vi "Fluxo automatico.vi"() -> ()   [LabVIEW 2011]
uses:
  <vilib>/Utility/error.llb/DialogType.ctl
  <vilib>/Analysis/6fits.llb/Curve Fitting Criteria.ctl
  <vilib>/DAQmx/write.llb/DAQmx Write (Digital Bool 1Line 1Point).vi
  <vilib>/DAQmx/create/channels.llb/DAQmx Create Channel (DO-Digital Output).vi
  <vilib>/DAQmx/miscellaneous.llb/DAQmx Fill In Error Info.vi
  <vilib>/Analysis/NI_AALPro.lvlib
panel:
  out "P-manual":dynamicdata(graph)
  in  "stop":bool
  in  "path":path=path "C:/H2_Painel/painel_auto/cinetica.txt"
  out "Polynomial Coefficients":dbl[](array[numeric])
  in  "STOP carga":dbl=5.0
  out "error":i32
  out "intercept":dbl
  out "slope":dbl
  in  "Def P":dbl
  in  "SET number":i32
  out "Linear Model Graph":dbl[][](graph)
  in  "N fit":i32
  in  "precision (6)":i16=3
  out "T":bool
  out "ZPit":bool
  out "Pit":bool
  out "Pf2":bool
  out "ZPf2":bool
  out "String_cinetica":string
  in  "wait vacuo":u32=30000
  in  "ATM wait":u32
  out "Thermometer":dbl(slide) scale=0.0..30.0
  out "String":string
  out "Camara":dbl(slide) scale=0.0..20.0 scale format="%#_3g"
  out "Vácuo":bool
  out "Atm":bool
  out "Câmara":bool
  out "Vol Ref":dbl(slide) scale=0.0..10.0 scale format="%#_4f"
  out "Entrada gás":bool
  # "P vol ref"
  # "P Câmara"
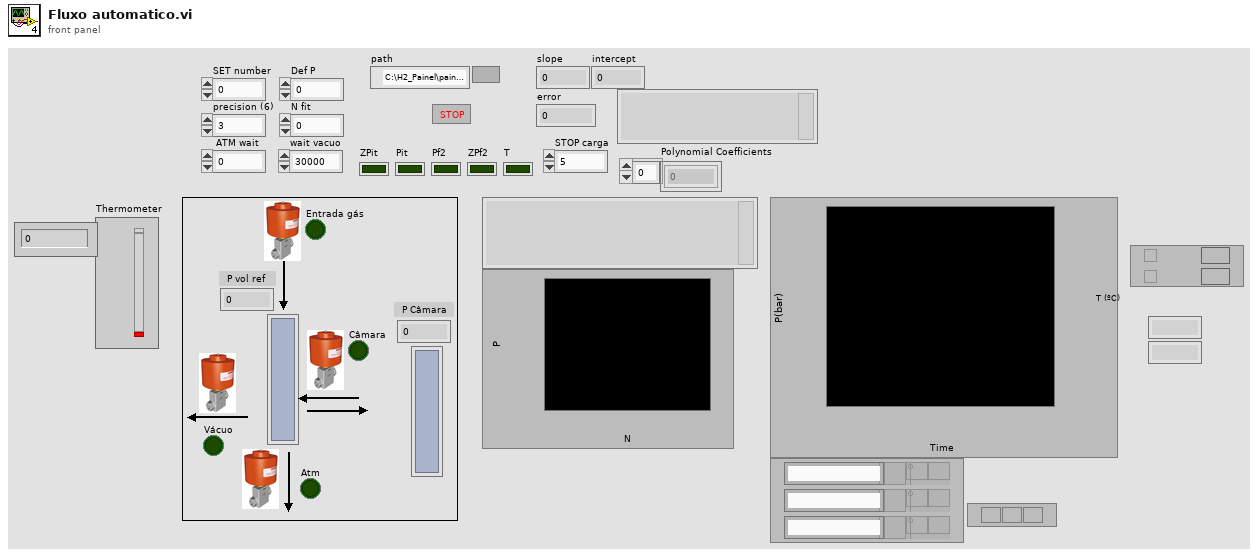
[diagram p1: front panel]
types:
  T1 = enum16{"open", "replace", "create", "open or create", "replace or create", "replace or create with confirmation"}
  T2 = typedef "DialogType.ctl" = u16
  T3 = typedef "NI_AALPro.lvlib/Curve Fitting Criteria.ctl" = u16
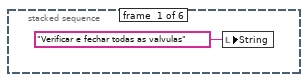
[diagram p2: hidden frame]
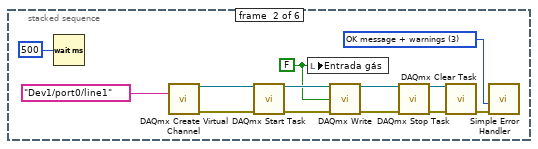
[diagram p3: hidden frame]
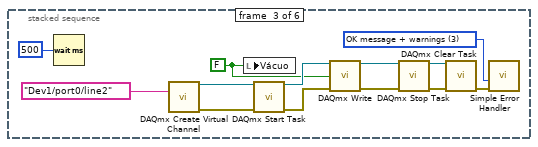
[diagram p4: hidden frame]
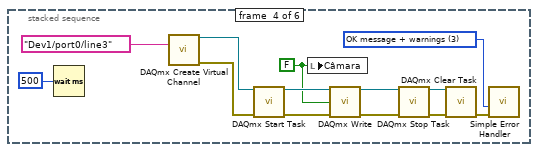
[diagram p5: hidden frame]
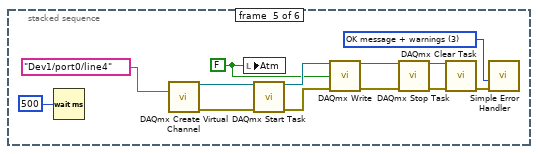
[diagram p6: hidden frame]
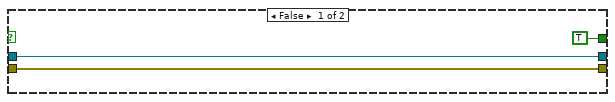
[diagram p8: hidden frame]
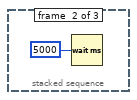
[diagram p9: hidden frame]
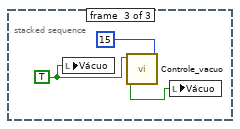
[diagram p10: hidden frame]
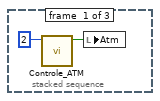
[diagram p11: hidden frame]
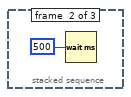
[diagram p12: hidden frame]
diagram:
  n1 = call "Read P T.vi"() -> ("P Set 2 Output 2"=w5:dbl, "T Set 2 Output"=w1:dbl)  [unwired: 4 in, 6 out]
  n2 = flat-sequence {
    frame #0 {
      w9 = FALSE ("Pit")
      "Pf2" <- w9
      "Pit" <- w9
      "ZPit" <- w9
      "ZPf2" <- w9
      "T" <- w9
    }
    frame #1 {
      n3 = stacked-sequence {
        frame #0 {
          n4 = local write "String"("Verificar e fechar todas as valvulas" ("String")) -> ()
        }
        frame #1 {
          w12 = FALSE ("Boolean 4")
          w17 = T2 3 items=["no dialog", "OK message", "continue or stop message", "OK message + warnings", "continue/stop + warnings"] ("type of dialog (OK msg:1)")
          n5 = Wait (ms)(milliseconds to wait=u32 500) -> ()  [unwired: 1 out]
          n6 = call-poly <vilib>:"DAQmx Create Virtual Channel.vi"("lines"=tag "Dev1/port0/line1") -> ("task out"=w15:refnum<k21>, "error out"=w16:errorcluster)  [unwired: 13 in]
          n7 = call <vilib>:"DAQmx Start Task.vi"("task/channels in"=w15, "error in"=w16) -> ("task out"=w18:refnum<k21>, "error out"=w19:errorcluster)  [unwired: 12 in]
          n8 = local write "Entrada gás"(w12) -> ()
          n9 = call-poly <vilib>:"DAQmx Write.vi"("task/channels in"=w18, "data"=w12, "error in"=w19) -> ("task out"=w23:refnum<k21>, "error out"=w20:errorcluster)  [unwired: 10 in, 1 out]
          n10 = call <vilib>:"DAQmx Stop Task.vi"("task/channels in"=w23, "error in"=w20) -> ("task out"=w22:refnum<k21>, "error out"=w21:errorcluster)  [unwired: 12 in]
          n11 = call <vilib>:"DAQmx Clear Task.vi"("task in"=w22, "error in"=w21) -> ("error out"=w14:errorcluster)  [unwired: 13 in]
          n12 = call <vilib>:"Simple Error Handler.vi"("type of dialog (OK msg:1)"=w17, "error in (no error)"=w14) -> ()  [unwired: 3 in, 5 out]
        }
        frame #2 {
          w25 = FALSE ("Boolean 4")
          w30 = T2 3 items=["no dialog", "OK message", "continue or stop message", "OK message + warnings", "continue/stop + warnings"] ("type of dialog (OK msg:1)")
          n13 = Wait (ms)(milliseconds to wait=u32 500) -> ()  [unwired: 1 out]
          n14 = call-poly <vilib>:"DAQmx Create Virtual Channel.vi"("lines"=tag "Dev1/port0/line2") -> ("task out"=w28:refnum<k21>, "error out"=w29:errorcluster)  [unwired: 13 in]
          n15 = local write "Vácuo"(w25) -> ()
          n16 = call <vilib>:"DAQmx Start Task.vi"("task/channels in"=w28, "error in"=w29) -> ("task out"=w31:refnum<k21>, "error out"=w32:errorcluster)  [unwired: 12 in]
          n17 = call-poly <vilib>:"DAQmx Write.vi"("task/channels in"=w31, "data"=w25, "error in"=w32) -> ("task out"=w36:refnum<k21>, "error out"=w33:errorcluster)  [unwired: 10 in, 1 out]
          n18 = call <vilib>:"DAQmx Stop Task.vi"("task/channels in"=w36, "error in"=w33) -> ("task out"=w35:refnum<k21>, "error out"=w34:errorcluster)  [unwired: 12 in]
          n19 = call <vilib>:"DAQmx Clear Task.vi"("task in"=w35, "error in"=w34) -> ("error out"=w27:errorcluster)  [unwired: 13 in]
          n20 = call <vilib>:"Simple Error Handler.vi"("type of dialog (OK msg:1)"=w30, "error in (no error)"=w27) -> ()  [unwired: 3 in, 5 out]
        }
        frame #3 {
          w38 = FALSE ("Boolean 4")
          w43 = T2 3 items=["no dialog", "OK message", "continue or stop message", "OK message + warnings", "continue/stop + warnings"] ("type of dialog (OK msg:1)")
          n21 = Wait (ms)(milliseconds to wait=u32 500) -> ()  [unwired: 1 out]
          n22 = call-poly <vilib>:"DAQmx Create Virtual Channel.vi"("lines"=tag "Dev1/port0/line3") -> ("task out"=w41:refnum<k21>, "error out"=w42:errorcluster)  [unwired: 13 in]
          n23 = call <vilib>:"DAQmx Start Task.vi"("task/channels in"=w41, "error in"=w42) -> ("task out"=w44:refnum<k21>, "error out"=w45:errorcluster)  [unwired: 12 in]
          n24 = local write "Câmara"(w38) -> ()
          n25 = call-poly <vilib>:"DAQmx Write.vi"("task/channels in"=w44, "data"=w38, "error in"=w45) -> ("task out"=w49:refnum<k21>, "error out"=w46:errorcluster)  [unwired: 10 in, 1 out]
          n26 = call <vilib>:"DAQmx Stop Task.vi"("task/channels in"=w49, "error in"=w46) -> ("task out"=w48:refnum<k21>, "error out"=w47:errorcluster)  [unwired: 12 in]
          n27 = call <vilib>:"DAQmx Clear Task.vi"("task in"=w48, "error in"=w47) -> ("error out"=w40:errorcluster)  [unwired: 13 in]
          n28 = call <vilib>:"Simple Error Handler.vi"("type of dialog (OK msg:1)"=w43, "error in (no error)"=w40) -> ()  [unwired: 3 in, 5 out]
        }
        frame #4 {
          w51 = FALSE ("Boolean 4")
          w56 = T2 3 items=["no dialog", "OK message", "continue or stop message", "OK message + warnings", "continue/stop + warnings"] ("type of dialog (OK msg:1)")
          n29 = Wait (ms)(milliseconds to wait=u32 500) -> ()  [unwired: 1 out]
          n30 = call-poly <vilib>:"DAQmx Create Virtual Channel.vi"("lines"=tag "Dev1/port0/line4") -> ("task out"=w54:refnum<k21>, "error out"=w55:errorcluster)  [unwired: 13 in]
          n31 = local write "Atm"(w51) -> ()
          n32 = call <vilib>:"DAQmx Start Task.vi"("task/channels in"=w54, "error in"=w55) -> ("task out"=w57:refnum<k21>, "error out"=w58:errorcluster)  [unwired: 12 in]
          n33 = call-poly <vilib>:"DAQmx Write.vi"("task/channels in"=w57, "data"=w51, "error in"=w58) -> ("task out"=w62:refnum<k21>, "error out"=w59:errorcluster)  [unwired: 10 in, 1 out]
          n34 = call <vilib>:"DAQmx Stop Task.vi"("task/channels in"=w62, "error in"=w59) -> ("task out"=w61:refnum<k21>, "error out"=w60:errorcluster)  [unwired: 12 in]
          n35 = call <vilib>:"DAQmx Clear Task.vi"("task in"=w61, "error in"=w60) -> ("error out"=w53:errorcluster)  [unwired: 13 in]
          n36 = call <vilib>:"Simple Error Handler.vi"("type of dialog (OK msg:1)"=w56, "error in (no error)"=w53) -> ()  [unwired: 3 in, 5 out]
        }
        frame #5 {
          n37 = Wait (ms)(milliseconds to wait=u32 3000) -> ()  [unwired: 1 out]
        }
      }
    }
    frame #2 {
      n38 = call "Read P T.vi"() -> ("P Set 2 Output 2"=w66:dbl)  [unwired: 4 in, 7 out]
      n39 = Multiply(x=w66, y=10.0) -> (x*y=w64:dbl)
      n40 = Greater?(x=w64, y=1.0) -> (0:w67:bool)
      n41 = flat-sequence {
        tunnel: w67 -> [w69]
        frame #0 {
          n42 = case shown="True" w69 {
            frame False {
            }
            frame True {
              n43 = call "Controle_ATM.vi"("seconds to wait"="ATM wait") -> ("String 2"=w72:string, "Atm"=w71:bool)  [unwired: 9 in]
              n44 = local write "Atm"(w71) -> ()
              n45 = local write "String"(w72) -> ()
            }
          }
        }
        frame #1 {
          n46 = Wait (ms)(milliseconds to wait=u32 5000) -> ()  [unwired: 1 out]
          n47 = local write "String"("Limpar volume referencia" ("String")) -> ()
        }
      }
    }
    frame #3 {
      w75 = TRUE ("Boolean")
      n48 = local write "Vácuo"(w75) -> ()
      n49 = call "Controle_vacuo.vi"("time (s) to wait vacuo"="wait vacuo", "Boolean"=w75) -> ("Vacuo"=w76:bool)  [unwired: 9 in]
      n50 = local write "Vácuo"(w76) -> ()
    }
    frame #4 {
      w90 = T3 2 items=["Least Square", "Least Absolute Residual", "Bisquare"] ("method")
      w82 = "\t"
      n51 = property on="N fit" class="DigNum (strict)"() -> ("Value"=w80:i32)  [unwired: 2 in, 2 out]
      n52 = for {
        N: w80 -> [_]
        tunnel: [w97] -> w86 mode=indexing
        tunnel: [w99] -> w91 mode=indexing
        i -> [w99]
        n53 = call "Read P T.vi"() -> ("P Set 2 Output 2"=w101:dbl)  [unwired: 4 in, 7 out]
        n54 = local write "String"("Ler ZPit" ("String")) -> ()
        n55 = Multiply(x=w101, y=10.0) -> (x*y=w97:dbl)
        n56 = local write "Vol Ref"(w97) -> ()
      }
      n57 = call <vilib>:"General Polynomial Fit.vi"("Y"=w86, "polynomial order"=0, "X"=w91, "method"=w90) -> ("Best Polynomial Fit"=w85:dbl[], "Polynomial Coefficients"=w88:dbl[])  [unwired: 8 in, 2 out]
      n58 = Build Array(w86, w85) -> (w84:dbl[][])
      n59 = property on="SET number" class="DigNum (strict)"() -> ("Value"=w83:i32)  [unwired: 2 in, 2 out]
      n60 = property on="precision (6)" class="DigNum (strict)"() -> ("Value"=w79:i16)  [unwired: 2 in, 2 out]
      n61 = Index Array(array=w88, index=0) -> (element=w87:dbl)
      n62 = local write "Linear Model Graph"(w84) -> ()
      n63 = Number To Decimal String(number=w83) -> (decimal integer string=w81:string)  [unwired: 1 in]
      n64 = Number To Fractional String(number=w87, precision (6)=w79) -> (F-format string=w96:string)  [unwired: 2 in]
      n65 = Concatenate Strings(w81, w82, w96, w82) -> (w93:string)
      n66 = property on="path" class="Path"() -> ("Value"=w78:path)  [unwired: 2 in, 2 out]
      n67 = flat-sequence {
        tunnel: [w105] -> w95
        tunnel: [w104] -> w94
        tunnel: w93 -> [w103]
        tunnel: w78 -> [w102]
        tunnel: w95 -> [w119]
        tunnel: w94 -> [w118]
        frame #0 {
          n68 = Open/Create/Replace File(file path (use dialog)=w102, operation (0:open)=T1."open") -> (refnum out=w111:refnum<file>, error out=w112:errorcluster)  [unwired: 2 in, 3 out]
          n69 = Set File Position(refnum=w111, from (0:start)=enum16{"start", "end", "current"}."end", error in=w112) -> (refnum out=w109:refnum<file>, error out=w108:errorcluster)  [unwired: 1 in]
          n70 = Write to Text File(file (use dialog)=w109, text=w103, error in=w108) -> (refnum out=w113:refnum<file>, error out=w114:errorcluster)  [unwired: 2 out]
          n71 = Close File(refnum=w113, error in=w114) -> (path=w105:path, error out=w106:errorcluster)
          n72 = call <vilib>:"Simple Error Handler.vi"("error in (no error)"=w106) -> ("error out"=w104:errorcluster)  [unwired: 1 in, 7 out]
        }
        frame #1 {
          n73 = local write "ZPit"(TRUE ("ZPit")) -> ()
          n74 = Wait (ms)(milliseconds to wait=u32 5000) -> ()  [unwired: 1 out]
          n75 = Read from Text File(file (use dialog)=w119, count=-1 ("Count  3"), error in=w118) -> (refnum out=w120:refnum<file>, text=w124:string, error out=w121:errorcluster)  [unwired: 1 in, 1 out]
          n76 = local write "String_cinetica"(w124) -> ()
          n77 = Close File(refnum=w120, error in=w121) -> (error out=w122:errorcluster)  [unwired: 1 out]
          n78 = local write "String"("abrir valvula entrada gas" ("String")) -> ()
          n79 = call <vilib>:"Simple Error Handler.vi"("error in (no error)"=w122) -> ()  [unwired: 1 in, 8 out]
        }
      }
    }
    frame #5 {
      n80 = while {
        tunnel: [w189] -> w127
        tunnel: [w188] -> w125
        stop <- w190 stop-if-true
        w202 = TRUE ("Boolean 4")
        n81 = call-poly <vilib>:"DAQmx Create Virtual Channel.vi"("lines"=tag "Dev1/port0/line1") -> ("task out"=w200:refnum<k21>, "error out"=w199:errorcluster)  [unwired: 13 in]
        n82 = call <vilib>:"DAQmx Start Task.vi"("task/channels in"=w200, "error in"=w199) -> ("task out"=w198:refnum<k21>, "error out"=w197:errorcluster)  [unwired: 12 in]
        n83 = local write "Entrada gás"(w202) -> ()
        n84 = call-poly <vilib>:"DAQmx Write.vi"("task/channels in"=w198, "data"=w202, "error in"=w197) -> ("task out"=w194:refnum<k21>, "error out"=w192:errorcluster)  [unwired: 10 in, 1 out]
        n85 = for {
          N: 1 -> [_]
          tunnel: [w208] -> w196
          tunnel: [w207] -> w195
          tunnel: w194 -> [w207]
          tunnel: [w206] -> w193
          tunnel: w192 -> [w206]
          n86 = call "Read P T.vi"() -> ("P Set 2 Output 2"=w210:dbl)  [unwired: 4 in, 7 out]
          n87 = Wait (ms)(milliseconds to wait=u32 5000) -> ()  [unwired: 1 out]
          n88 = Multiply(x=w210, y=10.0) -> (x*y=w205:dbl)
          n89 = local write "Vol Ref"(w205) -> ()
          n90 = Greater?(x=w205, y="Def P") -> (0:w208:bool)
        }
        n91 = case shown="True" w196 {
          tunnel: w195 -> [w212 w216]
          tunnel: w193 -> [w211 w215]
          tunnel: [TRUE FALSE] -> w190
          tunnel: [w212 _] -> w189
          tunnel: [w211 _] -> w188
          frame False {
          }
          frame True {
            n92 = flat-sequence {
              tunnel: w216 -> [w223]
              tunnel: w215 -> [w222]
              frame #0 {
                w224 = FALSE ("data")
                n93 = Wait (ms)(milliseconds to wait=u32 5000) -> ()  [unwired: 1 out]
                n94 = local write "Entrada gás"(w224) -> ()
                n95 = call-poly <vilib>:"DAQmx Write.vi"("task/channels in"=w223, "data"=w224, "error in"=w222) -> ("task out"=w219:refnum<k21>, "error out"=w218:errorcluster)  [unwired: 10 in, 1 out]
                n96 = call <vilib>:"DAQmx Stop Task.vi"("task/channels in"=w219, "error in"=w218) -> ("task out"=w221:refnum<k21>, "error out"=w220:errorcluster)  [unwired: 12 in]
                n97 = call <vilib>:"DAQmx Clear Task.vi"("task in"=w221, "error in"=w220) -> ()  [unwired: 13 in, 1 out]
              }
              frame #1 {
                n98 = stacked-sequence {
                  frame #0 {
                    n99 = call "Controle_ATM.vi"("seconds to wait"=u32 2) -> ("Atm"=w226:bool)  [unwired: 9 in, 1 out]
                    n100 = local write "Atm"(w226) -> ()
                  }
                  frame #1 {
                    n101 = Wait (ms)(milliseconds to wait=u32 5000) -> ()  [unwired: 1 out]
                  }
                  frame #2 {
                    w229 = TRUE ("Vácuo")
                    n102 = local write "Vácuo"(w229) -> ()
                    n103 = call "Controle_vacuo.vi"("time (s) to wait vacuo"=u32 15, "Boolean"=w229) -> ("Vacuo"=w230:bool)  [unwired: 9 in]
                    n104 = local write "Vácuo"(w230) -> ()
                  }
                }
              }
            }
          }
        }
      }
      n105 = while {
        tunnel: [w182] -> w128
        tunnel: w127 -> [w182]
        tunnel: [w181] -> w126
        tunnel: w125 -> [w181]
        stop <- w183 stop-if-true
        n106 = call "Read P T.vi"() -> ("P Set 2 Output 2"=w187:dbl)  [unwired: 4 in, 7 out]
        n107 = Multiply(x=w187, y=10.0) -> (x*y=w185:dbl)
        n108 = property on="Def P" class="DigNum (strict)"() -> ("Value"=w184:dbl)  [unwired: 2 in, 2 out]
        n109 = Greater Or Equal?(x=w185, y=w184) -> (x >= y?=w183:bool)
      }
      n110 = flat-sequence {
        tunnel: w128 -> [w132]
        tunnel: w126 -> [w131]
        frame #0 {
          w133 = FALSE ("Entrada gás")
          n111 = local write "Entrada gás"(w133) -> ()
          n112 = call-poly <vilib>:"DAQmx Write.vi"("task/channels in"=w132, "data"=w133, "error in"=w131) -> ("task out"=w130:refnum<k21>, "error out"=w135:errorcluster)  [unwired: 10 in, 1 out]
          n113 = call <vilib>:"DAQmx Stop Task.vi"("task/channels in"=w130, "error in"=w135) -> ("task out"=w129:refnum<k21>, "error out"=w134:errorcluster)  [unwired: 12 in]
          n114 = call <vilib>:"DAQmx Clear Task.vi"("task in"=w129, "error in"=w134) -> ()  [unwired: 13 in, 1 out]
        }
        frame #1 {
          n115 = Wait (ms)(milliseconds to wait=u32 5000) -> ()  [unwired: 1 out]
        }
        frame #2 {
          w142 = T3 2 items=["Least Square", "Least Absolute Residual", "Bisquare"] ("method")
          n116 = property on="N fit" class="DigNum (strict)"() -> ("Value"=w150:i32)  [unwired: 2 in, 2 out]
          n117 = for {
            N: w150 -> [_]
            tunnel: [w154] -> w146 mode=indexing
            tunnel: [w156] -> w141 mode=indexing
            i -> [w156]
            n118 = call "Read P T.vi"() -> ("P Set 2 Output 2"=w158:dbl)  [unwired: 4 in, 7 out]
            n119 = local write "String"("Ler ZPit" ("String")) -> ()
            n120 = Multiply(x=w158, y=10.0) -> (x*y=w154:dbl)
            n121 = local write "Vol Ref"(w154) -> ()
          }
          n122 = call <vilib>:"General Polynomial Fit.vi"("Y"=w146, "polynomial order"=0, "X"=w141, "method"=w142) -> ("Best Polynomial Fit"=w147:dbl[], "Polynomial Coefficients"=w144:dbl[])  [unwired: 8 in, 2 out]
          n123 = Build Array(w146, w147) -> (w148:dbl[][])
          n124 = property on="precision (6)" class="DigNum (strict)"() -> ("Value"=w151:i16)  [unwired: 2 in, 2 out]
          n125 = Index Array(array=w144, index=0) -> (element=w145:dbl)
          n126 = local write "Linear Model Graph"(w148) -> ()
          n127 = Number To Fractional String(number=w145, precision (6)=w151) -> (F-format string=w138:string)  [unwired: 2 in]
          n128 = Concatenate Strings(w138, "\t") -> (w139:string)
          n129 = property on="path" class="Path"() -> ("Value"=w137:path)  [unwired: 2 in, 2 out]
          n130 = flat-sequence {
            tunnel: [w162] -> w153
            tunnel: [w161] -> w152
            tunnel: w139 -> [w160]
            tunnel: w137 -> [w159]
            tunnel: w153 -> [w175]
            tunnel: w152 -> [w174]
            frame #0 {
              n131 = Open/Create/Replace File(file path (use dialog)=w159, operation (0:open)=T1."open") -> (refnum out=w168:refnum<file>, error out=w169:errorcluster)  [unwired: 2 in, 3 out]
              n132 = Set File Position(refnum=w168, from (0:start)=enum16{"start", "end", "current"}."end", error in=w169) -> (refnum out=w166:refnum<file>, error out=w165:errorcluster)  [unwired: 1 in]
              n133 = Write to Text File(file (use dialog)=w166, text=w160, error in=w165) -> (refnum out=w170:refnum<file>, error out=w171:errorcluster)  [unwired: 2 out]
              n134 = Close File(refnum=w170, error in=w171) -> (path=w162:path, error out=w163:errorcluster)
              n135 = call <vilib>:"Simple Error Handler.vi"("error in (no error)"=w163) -> ("error out"=w161:errorcluster)  [unwired: 1 in, 7 out]
            }
            frame #1 {
              n136 = local write "Pit"(TRUE ("ZPit")) -> ()
              n137 = Read from Text File(file (use dialog)=w175, count=-1 ("Count  3"), error in=w174) -> (refnum out=w176:refnum<file>, text=w180:string, error out=w177:errorcluster)  [unwired: 1 in, 1 out]
              n138 = local write "String_cinetica"(w180) -> ()
              n139 = Close File(refnum=w176, error in=w177) -> (error out=w178:errorcluster)  [unwired: 1 out]
              n140 = call <vilib>:"Simple Error Handler.vi"("error in (no error)"=w178) -> ()  [unwired: 1 in, 8 out]
              n141 = local write "String"("abrir valvula para camara" ("String")) -> ()
            }
          }
        }
      }
    }
    frame #6 {
      w232 = TRUE ("Boolean")
      w245 = T2 3 items=["no dialog", "OK message", "continue or stop message", "OK message + warnings", "continue/stop + warnings"] ("type of dialog (OK msg:1)")
      n142 = call-poly <vilib>:"DAQmx Create Virtual Channel.vi"("lines"=tag "Dev1/port0/line3") -> ("task out"=w247:refnum<k21>, "error out"=w246:errorcluster)  [unwired: 13 in]
      n143 = call <vilib>:"DAQmx Start Task.vi"("task/channels in"=w247, "error in"=w246) -> ("task out"=w244:refnum<k21>, "error out"=w243:errorcluster)  [unwired: 12 in]
      n144 = local write "Câmara"(w232) -> ()
      n145 = call-poly <vilib>:"DAQmx Write.vi"("task/channels in"=w244, "data"=w232, "error in"=w243) -> ("task out"=w237:refnum<k21>, "error out"=w234:errorcluster)  [unwired: 10 in, 1 out]
      n146 = while {
        tunnel: [FALSE ("Boolean")] -> w231
        tunnel: [w265] -> w236
        tunnel: w237 -> [w265]
        tunnel: [w264] -> w235
        tunnel: w234 -> [w264]
        stop <- w262 stop-if-true
        w255 = T3 0 items=["Least Square", "Least Absolute Residual", "Bisquare"] ("method")
        n147 = property on="N fit" class="DigNum (strict)"() -> ("Value"=w261:i32)  [unwired: 2 in, 2 out]
        n148 = for {
          N: w261 -> [_]
          tunnel: [w267] -> w254 mode=indexing
          tunnel: [w269] -> w253 mode=indexing
          i -> [w269]
          n149 = call "Read P T.vi"() -> ("P Set 2 Output 2"=w270:dbl)  [unwired: 4 in, 7 out]
          n150 = Multiply(x=w270, y=10.0) -> (x*y=w267:dbl)
          n151 = local write "Vol Ref"(w267) -> ()
        }
        n152 = call <vilib>:"Linear Fit.vi"("Y"=w254, "X"=w253, "method"=w255) -> ("Best Linear Fit"=w260:dbl[], "slope"=w249:dbl, "intercept"=→"intercept":dbl, "error"=→"error":i32)  [unwired: 8 in, 1 out]
        "slope" <- w249
        n153 = call <vilib>:"General Polynomial Fit.vi"("Y"=w254, "polynomial order"=0, "X"=w253, "method"=w255) -> ("Best Polynomial Fit"=w252:dbl[], "Polynomial Coefficients"=→"Polynomial Coefficients":dbl[])  [unwired: 8 in, 2 out]
        n154 = Absolute Value(x=w249) -> (abs(x)=w250:dbl)
        n155 = Build Array(w254, w260, w252) -> (w257:dbl[][])
        n156 = local write "Linear Model Graph"(w257) -> ()
        n157 = Less Or Equal?(x=w250, y="STOP carga") -> (x <= y?=w262:bool)
      }
      n158 = local write "Câmara"(w231) -> ()
      n159 = call-poly <vilib>:"DAQmx Write.vi"("task/channels in"=w236, "data"=w231, "timeout"=10.0, "error in"=w235) -> ("task out"=w240:refnum<k21>, "error out"=w239:errorcluster)  [unwired: 9 in, 1 out]
      n160 = call <vilib>:"DAQmx Stop Task.vi"("task/channels in"=w240, "error in"=w239) -> ("task out"=w241:refnum<k21>, "error out"=w242:errorcluster)  [unwired: 12 in]
      n161 = call <vilib>:"DAQmx Clear Task.vi"("task in"=w241, "error in"=w242) -> ("error out"=w248:errorcluster)  [unwired: 13 in]
      n162 = call <vilib>:"Simple Error Handler.vi"("type of dialog (OK msg:1)"=w245, "error in (no error)"=w248) -> ()  [unwired: 3 in, 5 out]
    }
    frame #7 {
      n163 = flat-sequence {
        frame #0 {
          n164 = Wait (ms)(milliseconds to wait=u32 5000) -> ()  [unwired: 1 out]
        }
        frame #1 {
          w277 = T3 2 items=["Least Square", "Least Absolute Residual", "Bisquare"] ("method")
          n165 = property on="N fit" class="DigNum (strict)"() -> ("Value"=w285:i32)  [unwired: 2 in, 2 out]
          n166 = for {
            N: w285 -> [_]
            tunnel: [w289] -> w281 mode=indexing
            tunnel: [w291] -> w276 mode=indexing
            i -> [w291]
            n167 = call "Read P T.vi"() -> ("P Set 2 Output 2"=w293:dbl)  [unwired: 4 in, 7 out]
            n168 = local write "String"("Ler Pf2" ("String")) -> ()
            n169 = Multiply(x=w293, y=10.0) -> (x*y=w289:dbl)
            n170 = local write "Vol Ref"(w289) -> ()
          }
          n171 = call <vilib>:"General Polynomial Fit.vi"("Y"=w281, "polynomial order"=0, "X"=w276, "method"=w277) -> ("Best Polynomial Fit"=w282:dbl[], "Polynomial Coefficients"=w279:dbl[])  [unwired: 8 in, 2 out]
          n172 = Build Array(w281, w282) -> (w283:dbl[][])
          n173 = property on="precision (6)" class="DigNum (strict)"() -> ("Value"=w286:i16)  [unwired: 2 in, 2 out]
          n174 = Index Array(array=w279, index=0) -> (element=w280:dbl)
          n175 = local write "Linear Model Graph"(w283) -> ()
          n176 = Number To Fractional String(number=w280, precision (6)=w286) -> (F-format string=w273:string)  [unwired: 2 in]
          n177 = Concatenate Strings(w273, "\t") -> (w274:string)
          n178 = property on="path" class="Path"() -> ("Value"=w272:path)  [unwired: 2 in, 2 out]
          n179 = flat-sequence {
            tunnel: [w297] -> w288
            tunnel: [w296] -> w287
            tunnel: w274 -> [w295]
            tunnel: w272 -> [w294]
            tunnel: w288 -> [w310]
            tunnel: w287 -> [w309]
            frame #0 {
              n180 = Open/Create/Replace File(file path (use dialog)=w294, operation (0:open)=T1."open") -> (refnum out=w303:refnum<file>, error out=w304:errorcluster)  [unwired: 2 in, 3 out]
              n181 = Set File Position(refnum=w303, from (0:start)=enum16{"start", "end", "current"}."end", error in=w304) -> (refnum out=w301:refnum<file>, error out=w300:errorcluster)  [unwired: 1 in]
              n182 = Write to Text File(file (use dialog)=w301, text=w295, error in=w300) -> (refnum out=w305:refnum<file>, error out=w306:errorcluster)  [unwired: 2 out]
              n183 = Close File(refnum=w305, error in=w306) -> (path=w297:path, error out=w298:errorcluster)
              n184 = call <vilib>:"Simple Error Handler.vi"("error in (no error)"=w298) -> ("error out"=w296:errorcluster)  [unwired: 1 in, 7 out]
            }
            frame #1 {
              n185 = local write "Pf2"(TRUE ("ZPit")) -> ()
              n186 = Read from Text File(file (use dialog)=w310, count=-1 ("Count  3"), error in=w309) -> (refnum out=w311:refnum<file>, text=w315:string, error out=w312:errorcluster)  [unwired: 1 in, 1 out]
              n187 = local write "String_cinetica"(w315) -> ()
              n188 = Close File(refnum=w311, error in=w312) -> (error out=w313:errorcluster)  [unwired: 1 out]
              n189 = call <vilib>:"Simple Error Handler.vi"("error in (no error)"=w313) -> ()  [unwired: 1 in, 8 out]
              n190 = local write "String"("abrir valvula para Atm -> vacuo" ("String")) -> ()
            }
          }
        }
      }
    }
    frame #8 {
      n191 = stacked-sequence {
        frame #0 {
          n192 = call "Controle_ATM.vi"("seconds to wait"=u32 2) -> ("Atm"=w317:bool)  [unwired: 9 in, 1 out]
          n193 = local write "Atm"(w317) -> ()
        }
        frame #1 {
          n194 = Wait (ms)(milliseconds to wait=u32 500) -> ()  [unwired: 1 out]
        }
        frame #2 {
          w320 = TRUE ("Vácuo")
          n195 = local write "Vácuo"(w320) -> ()
          n196 = property on="wait vacuo" class="DigNum (strict)"() -> ("Value"=w319:u32)  [unwired: 2 in, 2 out]
          n197 = call "Controle_vacuo.vi"("time (s) to wait vacuo"=w319, "Boolean"=w320) -> ("Vacuo"=w321:bool)  [unwired: 9 in]
          n198 = local write "Vácuo"(w321) -> ()
        }
      }
    }
    frame #9 {
      n199 = flat-sequence {
        frame #0 {
          n200 = Wait (ms)(milliseconds to wait=u32 1000) -> ()  [unwired: 1 out]
        }
        frame #1 {
          w332 = T3 2 items=["Least Square", "Least Absolute Residual", "Bisquare"] ("method")
          w333 = 0 ("polynomial order")
          n201 = property on="N fit" class="DigNum (strict)"() -> ("Value"=w343:i32)  [unwired: 2 in, 2 out]
          n202 = for {
            N: w343 -> [_]
            tunnel: [w347] -> w339 mode=indexing
            tunnel: [w349] -> w330 mode=indexing
            tunnel: [w346] -> w331 mode=indexing
            i -> [w349]
            n203 = call "Read P T.vi"() -> ("P Set 2 Output 2"=w351:dbl, "T Set 2 Output"=w346:dbl)  [unwired: 4 in, 6 out]
            n204 = local write "String"("Ler Zf2" ("String")) -> ()
            n205 = Multiply(x=w351, y=10.0) -> (x*y=w347:dbl)
            n206 = local write "Vol Ref"(w347) -> ()
          }
          n207 = call <vilib>:"General Polynomial Fit.vi"("Y"=w339, "polynomial order"=w333, "X"=w330, "method"=w332) -> ("Best Polynomial Fit"=w340:dbl[], "Polynomial Coefficients"=w337:dbl[])  [unwired: 8 in, 2 out]
          n208 = call <vilib>:"General Polynomial Fit.vi"("Y"=w331, "polynomial order"=w333, "X"=w330, "method"=w332) -> ("Polynomial Coefficients"=w327:dbl[])  [unwired: 8 in, 3 out]
          n209 = Index Array(array=w327) -> (element=w329:dbl)  [unwired: 1 in]
          n210 = Build Array(w339, w340) -> (w341:dbl[][])
          n211 = property on="precision (6)" class="DigNum (strict)"() -> ("Value"=w328:i16)  [unwired: 2 in, 2 out]
          n212 = Index Array(array=w337, index=0) -> (element=w338:dbl)
          n213 = local write "Linear Model Graph"(w341) -> ()
          n214 = Number To Fractional String(number=w338, precision (6)=w328) -> (F-format string=w334:string)  [unwired: 2 in]
          n215 = Number To Fractional String(number=w329, precision (6)=w328) -> (F-format string=w326:string)  [unwired: 2 in]
          n216 = Concatenate Strings(w334, "\t", w326, "\r\n") -> (w335:string)
          n217 = property on="path" class="Path"() -> ("Value"=w323:path)  [unwired: 2 in, 2 out]
          n218 = flat-sequence {
            tunnel: [w355] -> w345
            tunnel: [w354] -> w344
            tunnel: w335 -> [w353]
            tunnel: w323 -> [w352]
            tunnel: w345 -> [w368]
            tunnel: w344 -> [w367]
            tunnel: [w374] -> w324
            frame #0 {
              n219 = Open/Create/Replace File(file path (use dialog)=w352, operation (0:open)=T1."open") -> (refnum out=w361:refnum<file>, error out=w362:errorcluster)  [unwired: 2 in, 3 out]
              n220 = Set File Position(refnum=w361, from (0:start)=enum16{"start", "end", "current"}."end", error in=w362) -> (refnum out=w359:refnum<file>, error out=w358:errorcluster)  [unwired: 1 in]
              n221 = Write to Text File(file (use dialog)=w359, text=w353, error in=w358) -> (refnum out=w363:refnum<file>, error out=w364:errorcluster)  [unwired: 2 out]
              n222 = Close File(refnum=w363, error in=w364) -> (path=w355:path, error out=w356:errorcluster)
              n223 = call <vilib>:"Simple Error Handler.vi"("error in (no error)"=w356) -> ("error out"=w354:errorcluster)  [unwired: 1 in, 7 out]
            }
            frame #1 {
              w365 = TRUE ("ZPit")
              n224 = local write "T"(w365) -> ()
              n225 = local write "ZPf2"(w365) -> ()
              n226 = Read from Text File(file (use dialog)=w368, count=-1 ("Count  3"), error in=w367) -> (refnum out=w369:refnum<file>, text=w373:string, error out=w370:errorcluster)  [unwired: 1 in, 1 out]
              n227 = local write "String_cinetica"(w373) -> ()
              n228 = Close File(refnum=w369, error in=w370) -> (error out=w371:errorcluster)  [unwired: 1 out]
              n229 = call <vilib>:"Simple Error Handler.vi"("error in (no error)"=w371) -> ()  [unwired: 1 in, 8 out]
              n230 = local write "String"("abrir valvula para Atm -> vacuo" ("String")) -> ()
            }
            frame #2 {
              n231 = property on="SET number" class="DigNum (strict)"() -> ("Value"=w375:i32)  [unwired: 2 in, 2 out]
              n232 = Increment(x=w375) -> (x+1=w374:i32)
            }
          }
          n233 = local write "SET number"(w324) -> ()
        }
      }
    }
  }
  n234 = local write "ATM wait"(u32 1 ("ATM wait")) -> ()
  n235 = local write "wait vacuo"(u32 10 ("wait vacuo")) -> ()
  n236 = local write "N fit"(50 ("N fit")) -> ()
  n237 = local write "Thermometer"(w1) -> ()
  n238 = Multiply(x=w5, y=10.0) -> (x*y=w2:dbl)
  n239 = local write "Vol Ref"(w2) -> ()
  n240 = Merge Signals(w2, w1) -> (→"P-manual":dynamicdata)
